vi "Read Analogue.vi"(8 "error in (no error)":errorcluster, 11 "Analog Input in":refnum<class "Thermo Instrument.lvclass">) -> (0 "error out":errorcluster, 2 "Waveforms":waveform(dbl)[](array[waveform]), 3 "Analog Input out":refnum<class "Thermo Instrument.lvclass">)   [LabVIEW 2025, in "Thermo.lvlib" / "Thermo Instrument.lvclass"]
uses:
  Thermo Instrument.lvclass
  Thermo Instrument.lvclass/Thermo Instrument.ctl
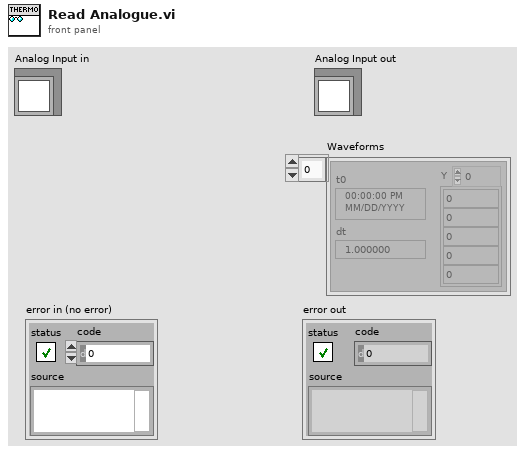
[diagram p1: front panel]
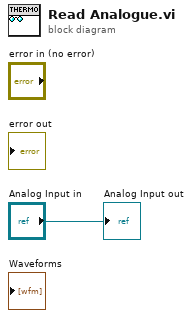
[diagram p0: block diagram]
diagram:
  "Analog Input out" <- "Analog Input in"
